vi "VMI_analyse_no_ref.vi"(0 "Peak Position Queue in":T1, 1 "Test Timing":bool, 9 "Image in":T1, 11 "Stop Button Ref":refnum<vi>, 12 "Image_array":i32[][](array[numeric]), 14 "Acquire Time":i32) -> (3 "Image_array out":i32[][](array[numeric]), 4 "Peaks Position Out":cluster{"X":sgl, "Y":sgl}[](array[cluster]), 6 "Current Image":T2(plugin-control), 10 "Peaks per frame":i32[](array[numeric]), 15 "error out":errorcluster)   [LabVIEW 2019]
uses:
  <vilib>/vision/Image Controls.llb/IMAQ Image.ctl
panel:
  out "x-y":u32
  out "size(s)":i32
  out "Single Image Points":cluster{"X":sgl, "Y":sgl}[](array[cluster])=[{"X"=212.6804, "Y"=106.63919}, {"X"=138.40689, "Y"=24.241379}, {"X"=316.33078, "Y"=38.515385}, {"X"=320.0, "Y"=56.301075}, {"X"=193.84746, "Y"=79.23729}, {"X"=195.92592, "Y"=104.85185}, {"X"=101.513275, "Y"=109.92921}, {"X"=345.82178, "Y"=117.28713}, {"X"=240.13792, "Y"=145.94827}, {"X"=10.357142, "Y"=157.24026}, {"X"=232.16667, "Y"=157.69608}, {"X"=104.34286, "Y"=174.28572}, {"X"=15.540541, "Y"=195.72298}, {"X"=93.1018, "Y"=207.8024}, {"X"=230.61539, "Y"=255.9011}, {"X"=129.26056, "Y"=275.0845}, {"X"=109.85714, "Y"=276.10715}, {"X"=46.11494, "Y"=281.16092}, {"X"=157.0, "Y"=298.7595}, {"X"=134.89635, "Y"=321.72562}]
  in  "Stop Button":bool
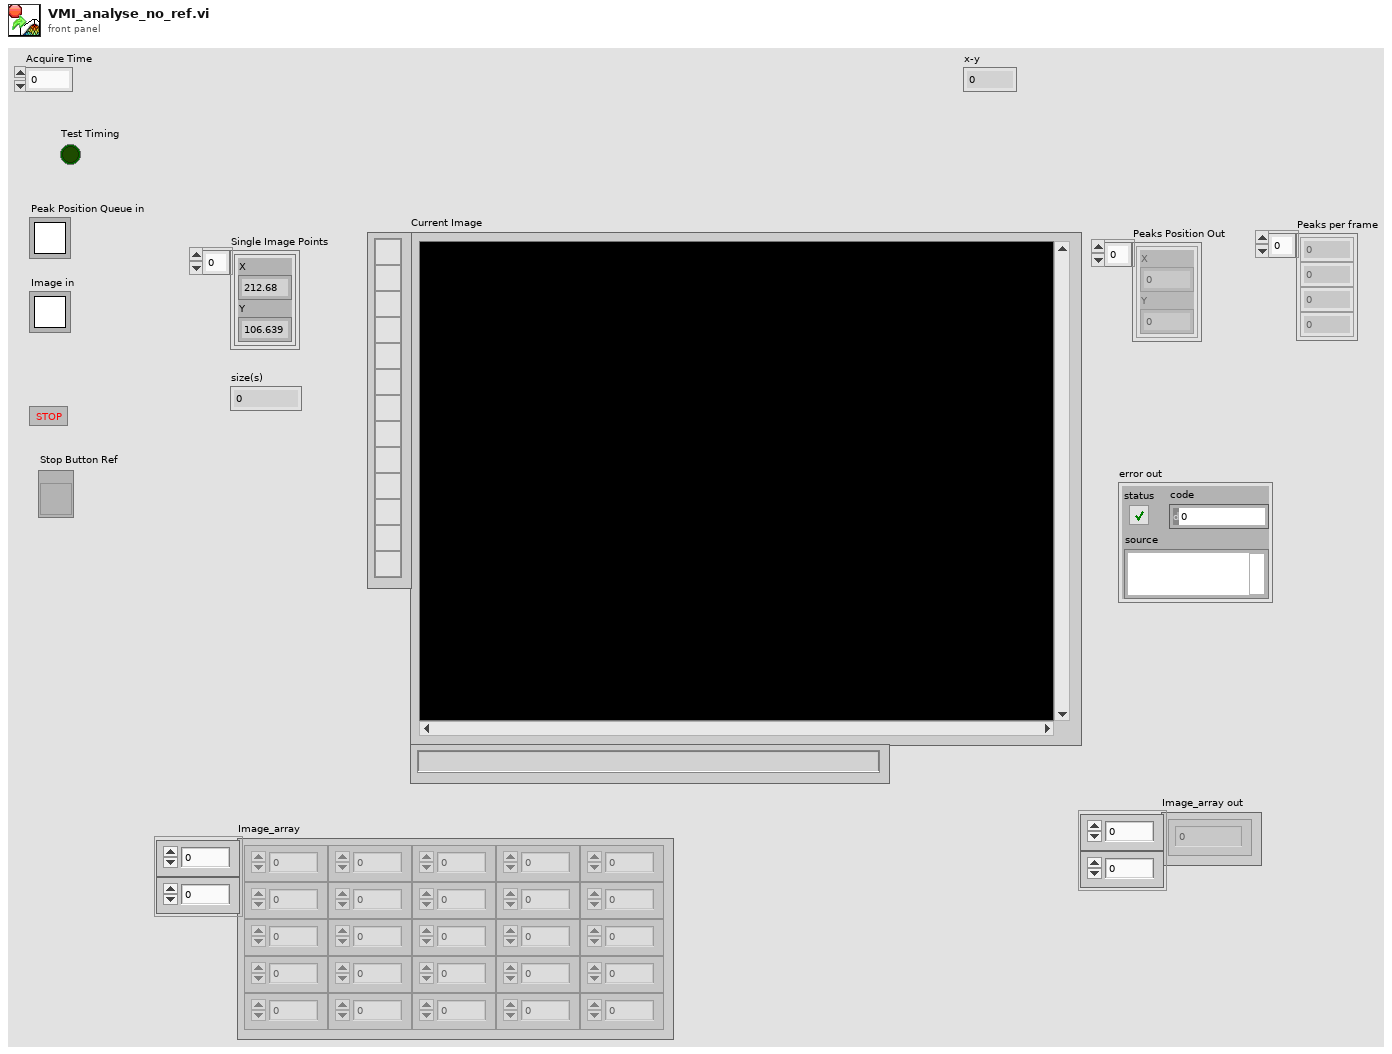
[diagram p1: front panel]
types:
  T1 = typedef "Queue RefNum" = refnum<k1>
  T2 = typedef "IMAQ Image.ctl" = refnum<image>
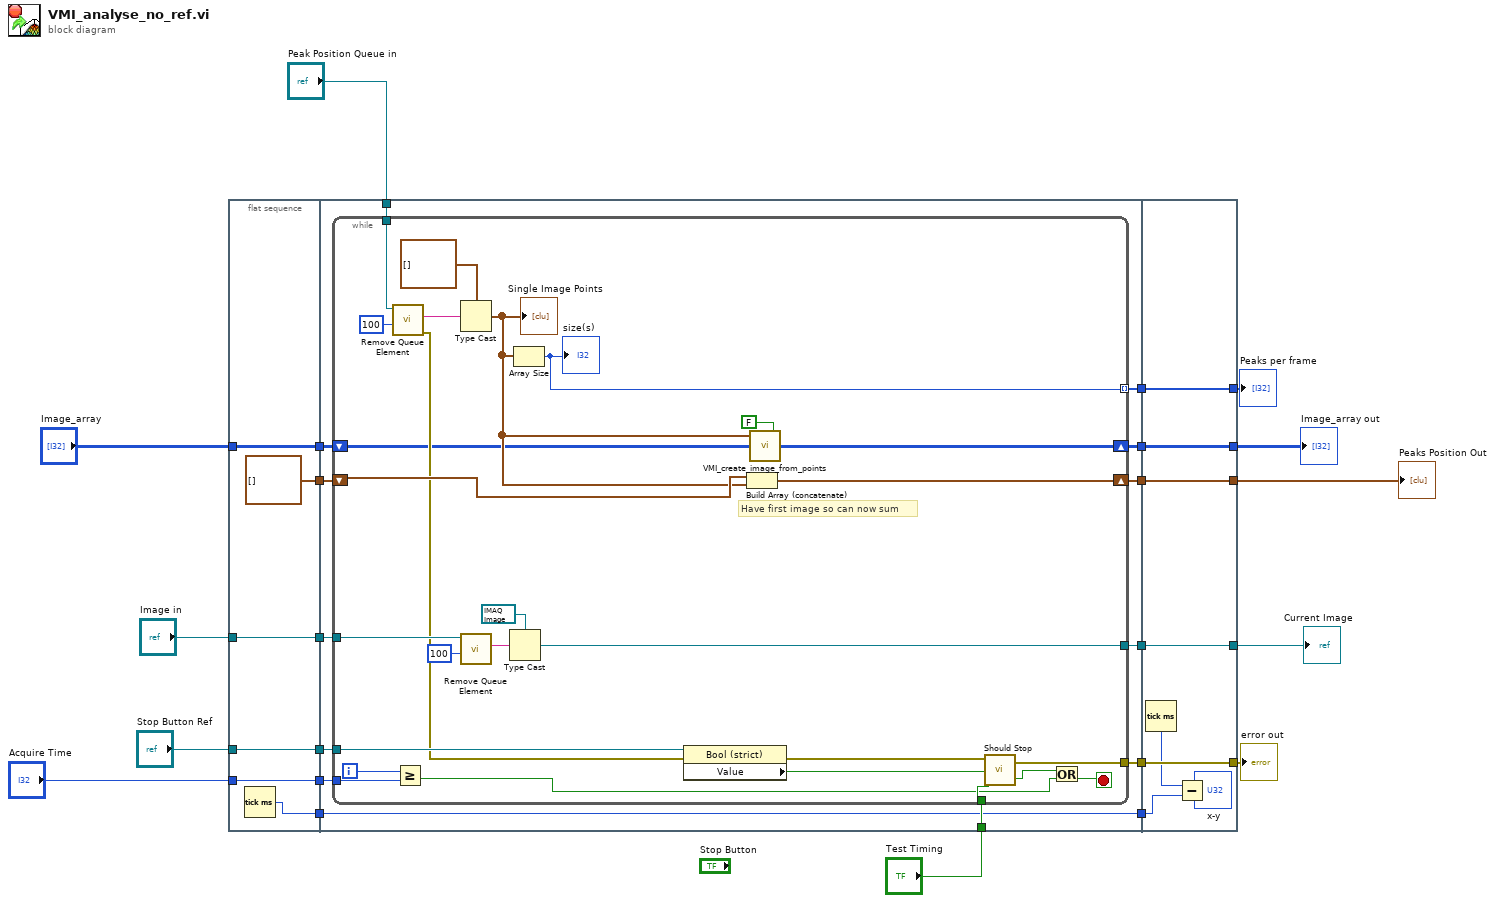
[diagram p0: block diagram]
diagram:
  n1 = flat-sequence {
    tunnel: "Acquire Time" -> [w27]
    tunnel: "Stop Button Ref" -> [w28]
    tunnel: "Image in" -> [w29]
    tunnel: [w29] -> w12
    tunnel: [w28] -> w11
    tunnel: [w27] -> w10
    tunnel: [w26] -> w8
    tunnel: [cluster{"X":sgl, "Y":sgl}[] []] -> w5
    tunnel: "Image_array" -> [w24]
    tunnel: [w24] -> w3
    tunnel: "Peak Position Queue in" -> [w40]
    tunnel: "Test Timing" -> [w37]
    tunnel: [w42] -> w15
    tunnel: [w39] -> w14
    tunnel: [w38] -> w13
    tunnel: w12 -> [w41]
    tunnel: w11 -> [w36]
    tunnel: w10 -> [w35]
    tunnel: [w34] -> w9
    tunnel: w8 -> [w34]
    tunnel: [w33] -> w7
    tunnel: w5 -> [w32]
    tunnel: [w31] -> w4
    tunnel: w3 -> [w30]
    tunnel: [w75] -> w19
    tunnel: [w76] -> w20
    tunnel: [w77] -> w23
    tunnel: w15 -> [w77]
    tunnel: w14 -> [w76]
    tunnel: w13 -> [w75]
    tunnel: w9 -> [w74]
    tunnel: w7 -> [w71]
    tunnel: [w71] -> w6
    tunnel: w4 -> [w70]
    tunnel: [w70] -> w1
    frame #0 {
      n2 = Tick Count (ms)() -> (millisecond timer value=w26:u32)
    }
    frame #1 {
      n3 = while {
        tunnel: w40 -> [w69]
        tunnel: w41 -> [w66]
        shift-right: [w63] -> w39
        shift-left: w32 -> [w62]
        tunnel: [w61] -> w42
        tunnel: [w60] -> w38 mode=indexing
        tunnel: w37 -> [w59]
        tunnel: w36 -> [w58]
        tunnel: w35 -> [w53]
        tunnel: [w47] -> w33
        shift-right: [w45] -> w31
        shift-left: w30 -> [w44]
        i -> [w54]
        stop <- w52 stop-if-true
        # "Have first image so can now sum"
        n4 = call <vilib>:"Remove Queue Element.vi"("ms timeout (-1)"=100, "queue"=w69) -> ("error out"=w56:errorcluster, "queue element"=w68:string)  [unwired: 4 in, 2 out]
        n5 = Greater Or Equal?(x=w54, y=w53) -> (x >= y?=w50:bool)
        n6 = Type Cast(type=cluster{"X":sgl, "Y":sgl}[] [], x=w68) -> (*(type *) &x=w46:cluster{"X":sgl, "Y":sgl}[])
        "Single Image Points" <- w46
        n7 = call <vilib>:"Remove Queue Element.vi"("ms timeout (-1)"=100, "queue"=w66) -> ("queue element"=w65:string)  [unwired: 4 in, 3 out]
        n8 = Type Cast(type=T2 refnum ("Image Out"), x=w65) -> (*(type *) &x=w47:T2)
        n9 = Array Size(array=w46) -> (size(s)=w60:i32)
        "size(s)" <- w60
        n10 = property class="Bool (strict)"(reference=w58, error in=w56) -> (error out=w55:errorcluster, "Value"=w57:bool)  [unwired: 1 out]
        n11 = Build Array (concatenate)(w62, w46) -> (w63:cluster{"X":sgl, "Y":sgl}[])
        n12 = call "VMI_create_image_from_points.vi"("New Array"=FALSE, "Input array"=w44, "Points"=w46) -> ("Image Array"=w45:i16[][])  [unwired: 2 in]
        n13 = call "Should Stop.vi"("error in 1"=w55, "Stop Button"=w57, "Look at Stop Button"=w59) -> ("error out"=w61:errorcluster, "Stop"=w51:bool)  [unwired: 2 in]
        n14 = Or(x=w51, y=w50) -> (x .or. y?=w52:bool)
      }
    }
    frame #2 {
      n15 = Tick Count (ms)() -> (millisecond timer value=w73:u32)
      n16 = Subtract(x=w73, y=w74) -> (x-y=→"x-y":u32)
    }
  }
  "error out" <- w23
  "Peaks Position Out" <- w20
  "Current Image" <- w6
  "Peaks per frame" <- w19
  "Image_array out" <- w1
